vi "fg_data_path.vi"(7 "fg_command":T1=enum."read", 8 "error in (no error)":errorcluster, 11 "path [] in":path[](array[path])) -> (0 "error out":errorcluster, 3 "path [] out":path[](array[path]))   [LabVIEW 2015, in "lv-bin.lvlib"]
uses:
  lv-bin.lvlib
  _controls/fg_command.ctl
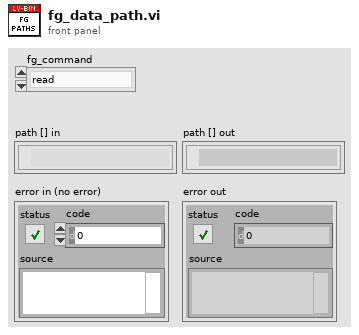
[diagram p1: front panel]
types:
  T1 = typedef "lv-bin.lvlib/fg_command.ctl" = enum16{"<fg_command>", "initialize", "read", "write", "shutdown", "<null>"}
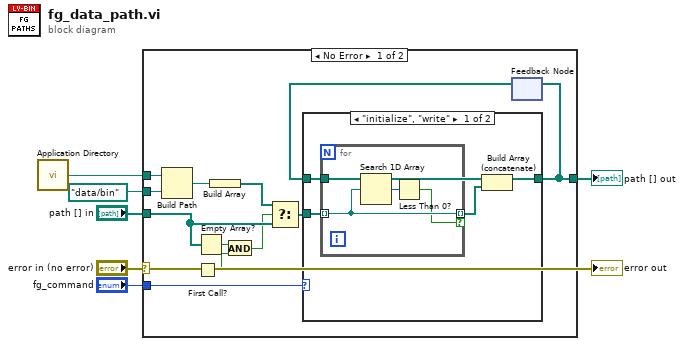
[diagram p0: block diagram]
diagram:
  n1 = call <vilib>:"Application Directory.vi"() -> ("Application Directory"=w2:path)
  n2 = case shown="No Error" "error in (no error)" {
    tunnel: [w18 _] -> w6
    tunnel: "fg_command" -> [w16 _]
    tunnel: "path [] in" -> [w15 _]
    tunnel: w2 -> [w13 _]
    tunnel: path "data/bin" ("Application Directory") -> [w12 _]
    frame No Error {
      n3 = Build Path(base path=w13, name or relative path=w12) -> (appended path=w9:path)
      n4 = First Call?() -> (First Call?: T/F=w7:bool)
      n5 = Empty Array?(array=w15) -> (empty?=w11:bool)
      n6 = Build Array(w9) -> (w10:path[])
      n7 = And(x=w11, y=w7) -> (x .and. y?=w8:bool)
      n8 = Select(t=w10, s=w8, f=w15) -> (s? t:f=w14:path[])
      n9 = feedback #1() -> (w17:path[])  [unwired: 1 in]
      n10 = case shown="\"initialize\", \"write\"" w16 {
        tunnel: w14 -> [w22 _]
        tunnel: [w20 w27] -> w18
        tunnel: w17 -> [w19 w27]
        frame "initialize", "write" {
          n11 = for {
            tunnel: w19 -> [w26]
            tunnel: w22 -> [w25] mode=indexing
            tunnel: [w25] -> w21 mode=indexing if=w24
            n12 = Search 1D Array(1D array=w26, element=w25) -> (index of element=w23:i32)  [unwired: 1 in]
            n13 = Less Than 0?(x=w23) -> (x < 0?=w24:bool)
          }
          n14 = Build Array (concatenate)(w19, w21) -> (w20:path[])
        }
        frame "read", Default {
        }
      }
      n15 = feedback-in #1(w18) -> ()
    }
    frame Error {
    }
  }
  "path [] out" <- w6
  "error out" <- "error in (no error)"
